vi "Explainations.vi"(11 "FRF":cluster{"x0":dbl, "df":dbl, dbl[]}[](graph)) -> ()   [LabVIEW 2022 SP3]
panel:
  in  "Typical Ranges":string[][](table)=[["   Mode(s)", "     Range", "   Average"], ["A0", "264-290 Hz", "276 Hz"], ["CBR", "380 – 420 Hz", "400 Hz"], ["B1-", "393-470 Hz", "444 Hz"], ["B1+", "473-593 Hz", "541 Hz"], ["Transition Hill", "800-1300 Hz", ""], ["Bridge Hill", "1750-3000 Hz", ""], ["Upper Hill", "3000-7000 Hz", ""]]
  # "Interpreting the FRF using Oberlin Terminology"
  # "Web links\nTalks: https://www.youtube.com/channel/UCb8nC_6JQtlqal0-bVQZMeg\nBooks:\nhttps://www.violinacoustics.com\nhttps://euphonics.org/homepage/"
  # "Signature Modes"
  # "Multiple Overlapping Modes"
  # "isotropic monopole radiation"
  # "increasingly directional multipole radiation"
  # "Upper Hill\n[vertical excitiation only]"
  # "Bridge Hill"
  # "Transition Hill"
  # "A0"
  # "CBR"
  # "B1-"
  # "B1+"
  # "G0"
  # "D0"
  # "A0"
  # "E0"
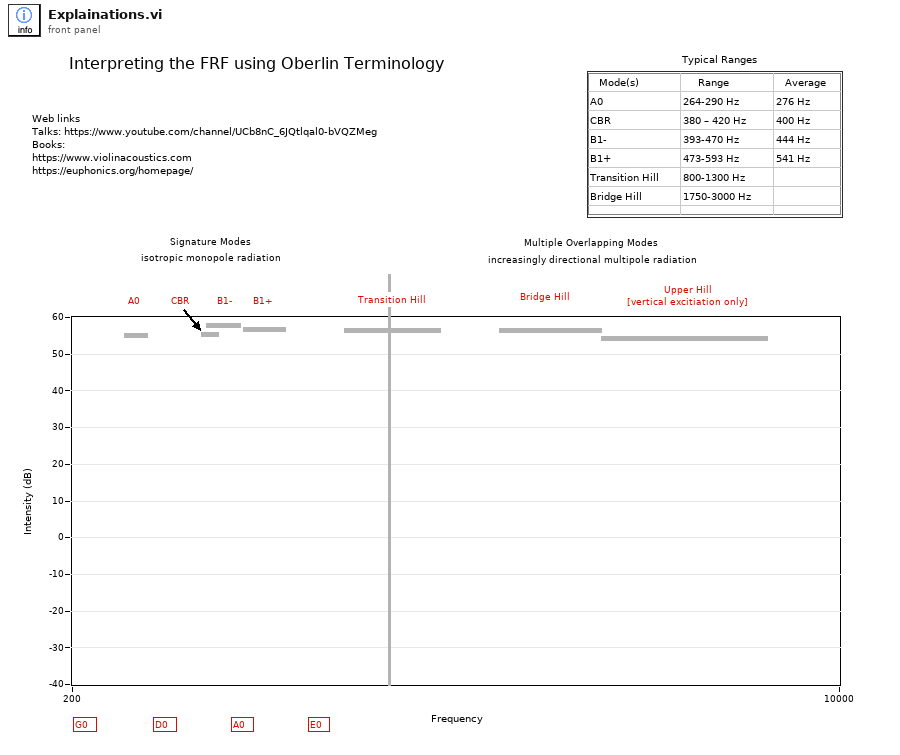
[diagram p1: front panel]
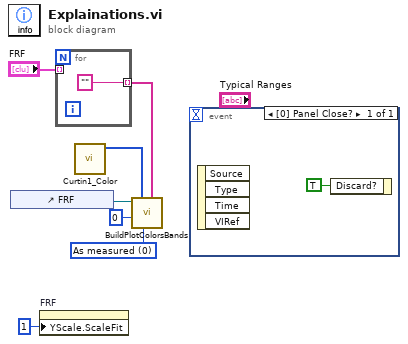
[diagram p0: block diagram]
diagram:
  w4 = u16 0 items=["As measured", "Normalize", "Separate", "Cplx Average", "Real Average"] ("View Type")
  n1 = control-ref of="FRF"() -> (w6:refnum<vi>)
  n2 = property on="FRF" class="WFGraph (strict)"("YScale.ScaleFit"=u8 1 ("Y Scale.Scale Fit")) -> ()  [unwired: 2 in, 2 out]
  n3 = for {
    tunnel: "FRF" -> [_] mode=indexing
    tunnel: [""] -> w1 mode=indexing
  }
  n4 = call "Curtin1_Color.vi"() -> ("Color palette"=w3:u32[])  [unwired: 10 in, 1 out]
  n5 = call "BuildPlotColorsBands.vi"("Labels"=w1, "View Type"=w4, "Colors"=w3, "Bands"=u16 0, "WaveformGraph in"=w6) -> ()  [unwired: 6 in, 1 out]
  n6 = event shown="[0] Panel Close?" {
    selector: _ -> [_]
    dyn-events: _ -> [_]
    timeout: _ -> [_]
    event Panel Close? {
      n7 = event-data() -> ()  [unwired: 1 in, 4 out]
      n8 = event-data("Discard?"=TRUE) -> ()  [unwired: 1 in, 1 out]
    }
  }
